vi "NXT Camera Test3.vi"() -> ()   [LabVIEW 2016]
uses:
  <vilib>/NXT/Block Support/NXT_InputPort.ctl
  <vilib>/NXT/Block Support/NXT_OutputPort.ctl
  <vilib>/NXT/NXTIO Xnodes/NXTIONodeSubVIs/NXTMoveMotors.vi
  <vilib>/NXT/NXTIO Xnodes/NXTIONodeSubVIs/NXTStopMotors.vi
  <vilib>/NXT/Subs/LVHSConnector.ctl
  <vilib>/NXT/NXTIO Xnodes/AddressXNode/NXTIOAddress.xnode
  <vilib>/NXT/NXTIO Xnodes/NXTIOXNode/NXTIO.xnode
  <vilib>/NXT/LegoClasses/BrickReference/BrickReference.lvclass
panel:
  in  "stop":bool
  out "Power":bool
  out "X Upper Left":u8
  out "X Lower Right":u8
  out "Y Lower Right":u8
  out "Y Upper Left":u8
  out "Count":u8
  out "Color":u8
  in  "Cluster":T1 {"Tracking Mode" items=["Disable Tracking", "Get First Object", "Get n th Object", "Enable Tracking", "Sort Objects  by size", "Sort Objects  by Colors", "Illumination on ", "Illumination Off", "Write Colormap", "Read Colormap", "Line tracking mode", "Object Tracking mode"]}
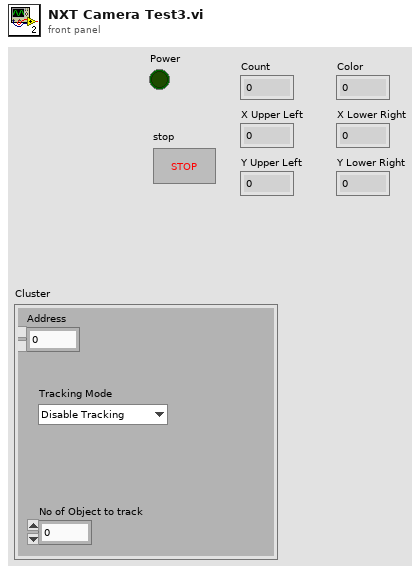
[diagram p1: front panel]
types:
  T1 = cluster{"Address":dbl, "No of Object to track":dbl, "Tracking Mode":u8}
  T2 = cluster{"Tracking Mode":u8, "Object Number to Track":u8, "Address":u8}
  T3 = typedef "NXT_InputPort.ctl" = u32
  T4 = typedef "LVHSConnector.ctl" = refnum<class "BrickReference.lvclass">
  T5 = cluster{"Total Tracked Objects":u8, "Color":u8, "X Upper Left":u8, "Y Upper Left":u8, "X Lower Right":u8, "Y Lower Right":u8, "Status (boolean)":bool}
  T6 = typedef "NXT_OutputPort.ctl" = u8
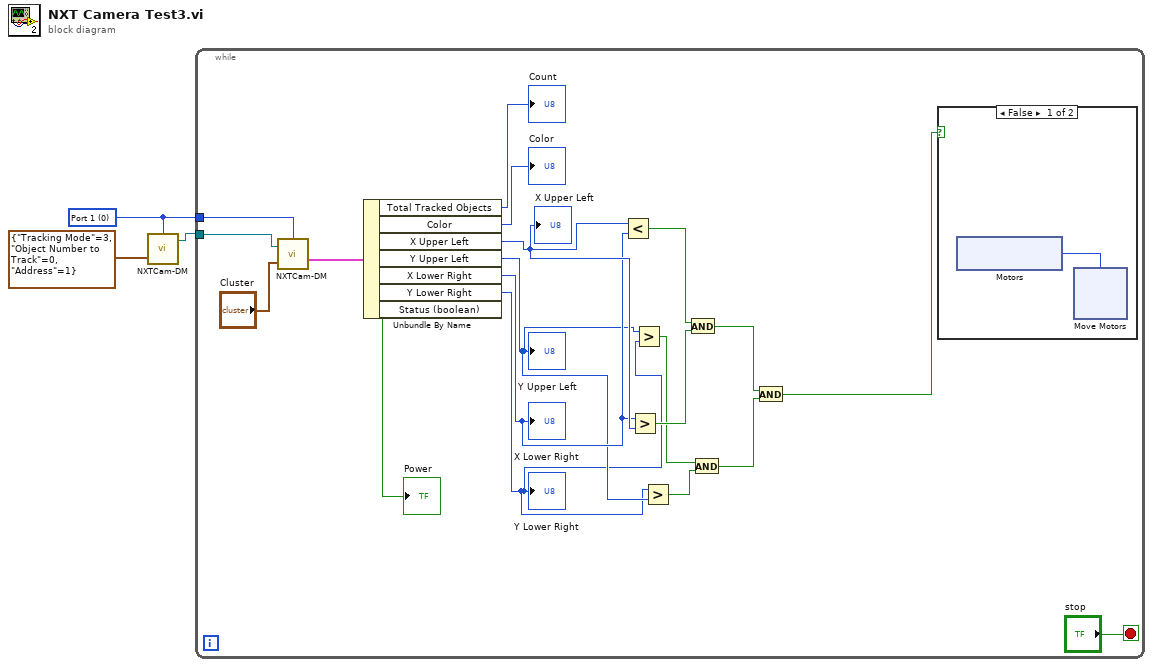
[diagram p0: block diagram]
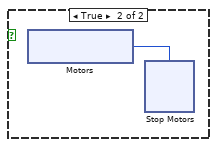
[diagram p2: hidden frame]
diagram:
  w1 = T3 0 items=["Port 1", "Port 2", "Port 3", "Port 4"] ("Input Port")
  n1 = call "NXTCam-DM.vi"("Input of NXTCam"=T2 {"Tracking Mode"=3, "Object Number to Track"=0, "Address"=1}, "Input Port"=w1) -> ("NXT dup"=w3:T4)  [unwired: 1 in, 1 out]
  n2 = while {
    tunnel: w1 -> [w16]
    tunnel: w3 -> [w15]
    stop <- "stop" stop-if-true
    n3 = call "NXTCam-DM.vi"("Input of NXTCam"="Cluster", "NXT"=w15, "Input Port"=w16) -> ("Output of NXTCam"=w17:T5)  [unwired: 1 out]
    n4 = Unbundle By Name(w17) -> ("Total Tracked Objects"=→"Count":u8, "Color"=→"Color":u8, "X Upper Left"=w14:u8, "Y Upper Left"=w10:u8, "X Lower Right"=w13:u8, "Y Lower Right"=w9:u8, "Status (boolean)"=→"Power":bool)
    "X Upper Left" <- w14
    "X Lower Right" <- w13
    "Y Lower Right" <- w9
    "Y Upper Left" <- w10
    n5 = Less?(x=w14, y=w13) -> (x < y?=w12:bool)
    n6 = Greater?(x=w13, y=w14) -> (0:w11:bool)
    n7 = Greater?(x=w10, y=w9) -> (0:w8:bool)
    n8 = Greater?(x=w9, y=w10) -> (0:w7:bool)
    n9 = And(x=w12, y=w11) -> (x .and. y?=w6:bool)
    n10 = And(x=w8, y=w7) -> (x .and. y?=w5:bool)
    n11 = And(x=w6, y=w5) -> (x .and. y?=w4:bool)
    n12 = case shown="False" w4 {
      frame False {
        n13 = xnode "Motors"() -> ("Motor"=w23:T6)
        n14 = xnode "Move Motors"("Motors"=w23) -> ()  [unwired: 2 in, 1 out]
      }
      frame True {
        n15 = xnode "Motors"() -> ("Motor"=w32:T6)
        n16 = xnode "Stop Motors"("Motors"=w32) -> ()  [unwired: 1 in, 1 out]
      }
    }
  }
